vi "gentec-M-Link.Get Head connected.vi"(0 "VISA resource In":refnum<visa-resource-name>, 5 "error in (no error)":errorcluster) -> (11 "Data Read":string, 13 "Read Timeout":bool, 14 "VISA resource Out":refnum<visa-resource-name>, 16 "Head connected?":bool, 19 "error out":errorcluster)   [LabVIEW 2014, in "gentec-M-Link - Driver.lvlib"]
doc: "Data to write: prb\n\nQueries the head connected flag. If no head is present the command does not reply. This allows the cojntrol software to periodically poll for a head connection. If 1 is replied, a head is connected; no reply means no head is connected."
uses:
  gentec-M-Link - Driver.lvlib
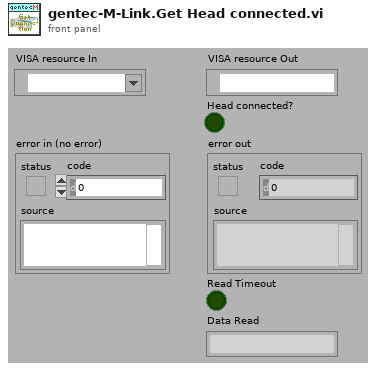
[diagram p1: front panel]
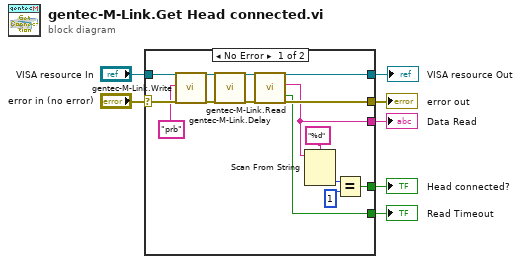
[diagram p0: block diagram]
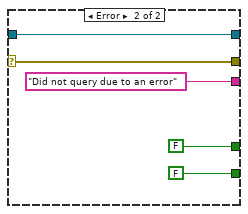
[diagram p2: hidden frame]
diagram:
  n1 = case shown="No Error" "error in (no error)" {
    selector: "error in (no error)" -> [w19 w27]
    tunnel: [w20 w27] -> w6
    tunnel: "VISA resource In" -> [w18 w26]
    tunnel: [w17 w26] -> w4
    tunnel: [w9 FALSE ("Found")] -> w3
    tunnel: [w12 "Did not query due to an error" ("Data Read")] -> w2
    tunnel: [w13 FALSE ("Read Timeout")] -> w1
    frame No Error {
      n2 = call "gentec-M-Link.Write.vi"("VISA resource (In)"=w18, "Data To Write"="prb", "error in (no error)"=w19) -> ("VISA resource (Out)"=w22:refnum<visa-resource-name>, "error out"=w21:errorcluster)  [unwired: 14 in, 1 out]
      n3 = call "gentec-M-Link.Delay.vi"("VISA resource In"=w22, "error in (no error)"=w21) -> ("VISA resource Out"=w16:refnum<visa-resource-name>, "error out"=w15:errorcluster)  [unwired: 16 in]
      n4 = call "gentec-M-Link.Read.vi"("VISA resource (In)"=w16, "error in (no error)"=w15) -> ("VISA resource (Out)"=w17:refnum<visa-resource-name>, "Data Read"=w12:string, "Read Timeout"=w13:bool, "error out"=w20:errorcluster)  [unwired: 13 in, 1 out]
      n5 = Scan From String(format string="%d", input string=w12) -> (output 1=w10:i32)  [unwired: 3 in, 3 out]
      n6 = Equal?(x=w10, y=1) -> (x = y?=w9:bool)
    }
    frame Error {
    }
  }
  "error out" <- w6
  "VISA resource Out" <- w4
  "Head connected?" <- w3
  "Data Read" <- w2
  "Read Timeout" <- w1
